vi "NMEA_PARSER.vi"(0 "previous partial sentence":string, 1 "sensor data":string, 3 "error in (no error)":errorcluster) -> (7 "remaining partial sentence":string, 8 "GPS data":T1 {"oldest read timestamp" format="%#_10g"; "latitude (deg)" format="%#_10g"; "longitude (deg)" format="%#_10g"}, 10 "error out":errorcluster)   [LabVIEW 2024]
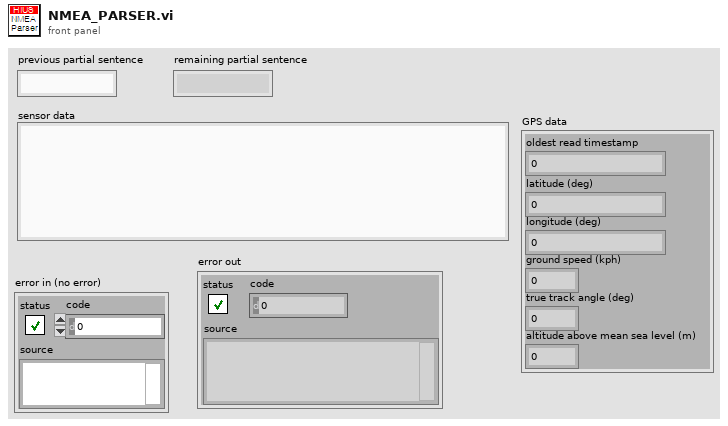
[diagram p1: front panel]
types:
  T1 = cluster{"oldest read timestamp":dbl, "latitude (deg)":dbl, "longitude (deg)":dbl, "ground speed (kph)":dbl, "true track angle (deg)":dbl, "altitude above mean sea level (m)":dbl}
  T2 = cluster{"oldest read timestamp":dbl, "latitude":dbl, "longitude":dbl, "speed over ground (kph)":dbl, "true track angle (deg)":dbl, "altitude above mean sea level":dbl}
  T3 = cluster{"time of fix":cluster{"included?":bool, "time (UTC)":dbl}, "status":cluster{"included?":bool, "value":u16}, "latitude":cluster{"included?":bool, "latitude (deg)":dbl}, "longitude":cluster{"included?":bool, "longitude (deg)":dbl}, "ground speed":cluster{"included?":bool, "speed (knots)":dbl}, "true track angle":cluster{"included?":bool, "angle (deg)":dbl}, "magnetic variation":cluster{"included?":bool, "variation (deg)":dbl}, "type of fix":cluster{"included?":bool, "mode":u16}}
  T4 = cluster{"time of fix":cluster{"included?":bool, "time (UTC)":dbl}, "latitude":cluster{"included?":bool, "latitude (deg)":dbl}, "longitude":cluster{"included?":bool, "longitude (deg)":dbl}, "ground speed (km/h)":cluster{"included?":bool, "speed (km/h)":dbl}, "ture track angle":cluster{"included?":bool, "angle (deg)":dbl}}
  T5 = cluster{"time of fix":cluster{"included?":bool, "time (UTC)":dbl}, "latitude":cluster{"included?":bool, "latitude (deg)":dbl}, "longitude":cluster{"included?":bool, "longitude (deg)":dbl}, "fix quality":cluster{"included?":bool, "quality":u16}, "number of satellites in view":cluster{"included?":bool, "number of satellites":i8}, "horizontal dilution of precision":cluster{"included?":bool, "horizontal DOP":dbl}, "altitude above mean sea level":cluster{"included?":bool, "altitude (m)":dbl}, "height of geoid above WGS84":cluster{"included?":bool, "height of geoid (m)":dbl}, "time since last DGPS update":cluster{"included?":bool, "time (s)":dbl}, "DGPS station ID number":cluster{"included?":bool, "station ID number":dbl}}
  T6 = cluster{"true track made good":cluster{"included?":bool, "true track made good (deg)":dbl}, "magnetic track made good":cluster{"included?":bool, "magnetic track made good (deg)":dbl}, "ground speed (knots)":cluster{"included?":bool, "speed (knots)":dbl}, "ground speed (km/h)":cluster{"included?":bool, "speed (km/h)":dbl}, "type of fix":cluster{"included?":bool, "mode":u16}}
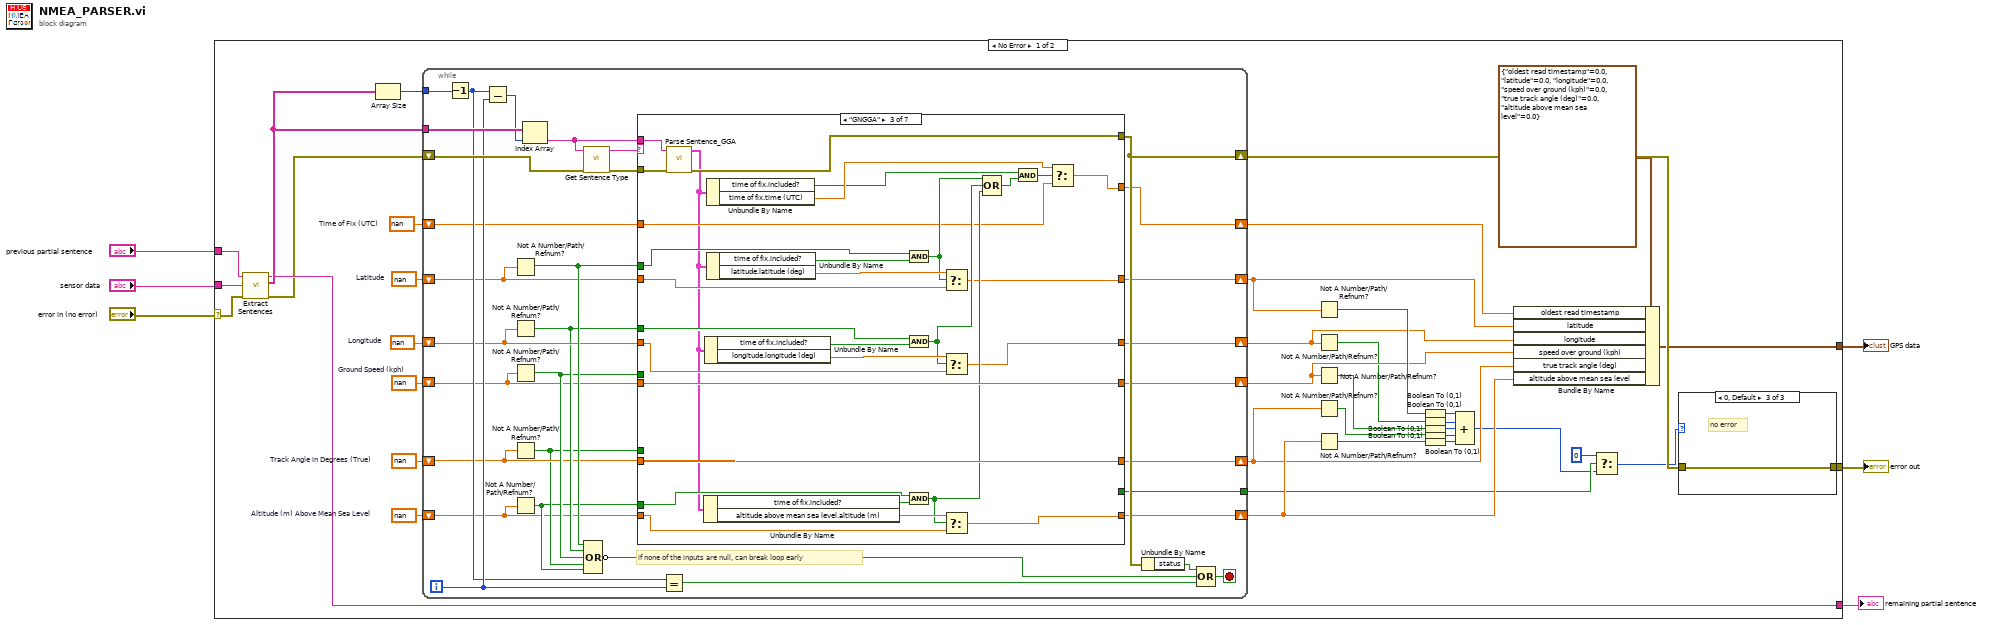
[diagram p0: block diagram]
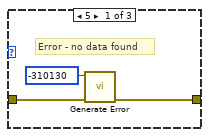
[diagram p2: hidden frame]
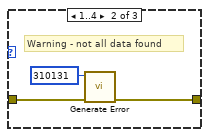
[diagram p3: hidden frame]
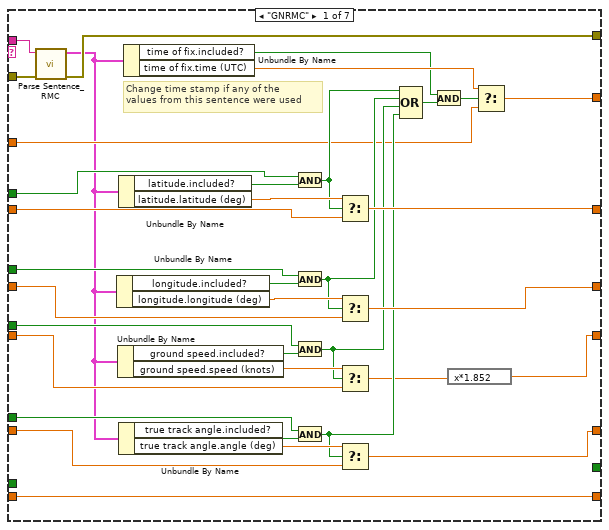
[diagram p4: hidden frame]
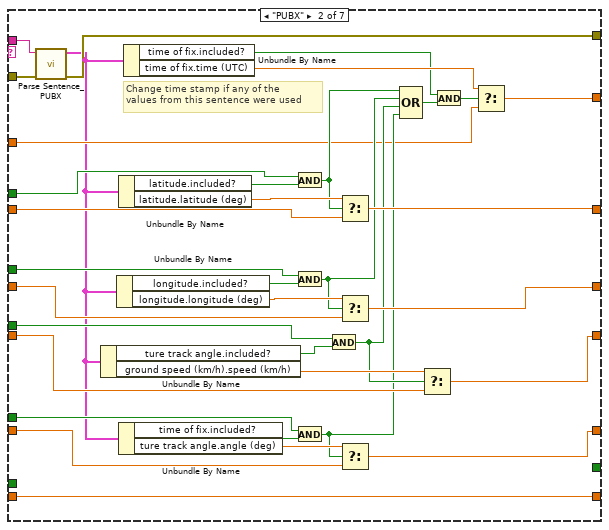
[diagram p5: hidden frame]
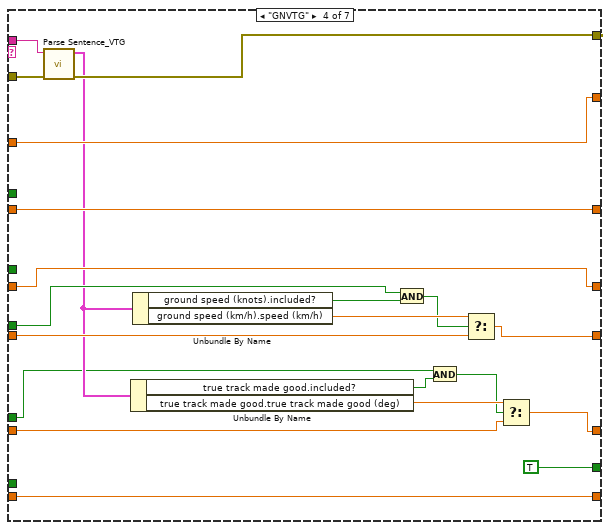
[diagram p6: hidden frame]
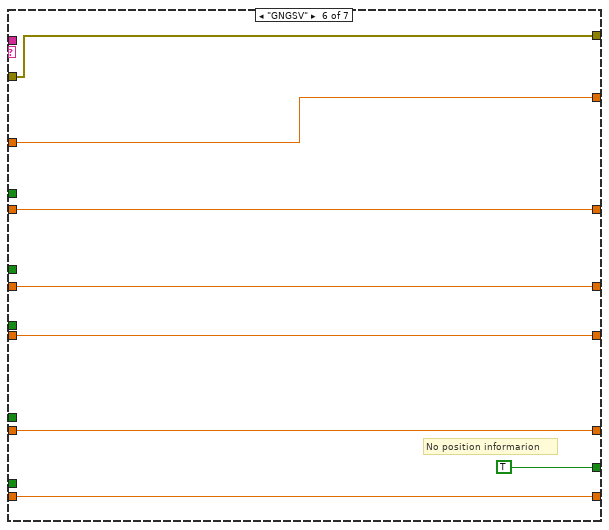
[diagram p8: hidden frame]
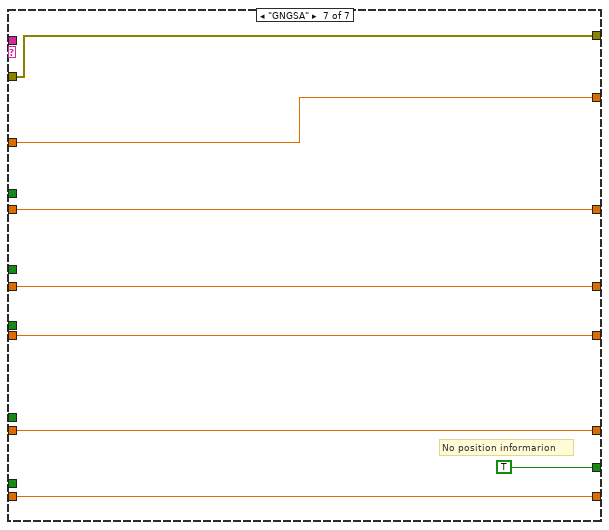
[diagram p9: hidden frame]
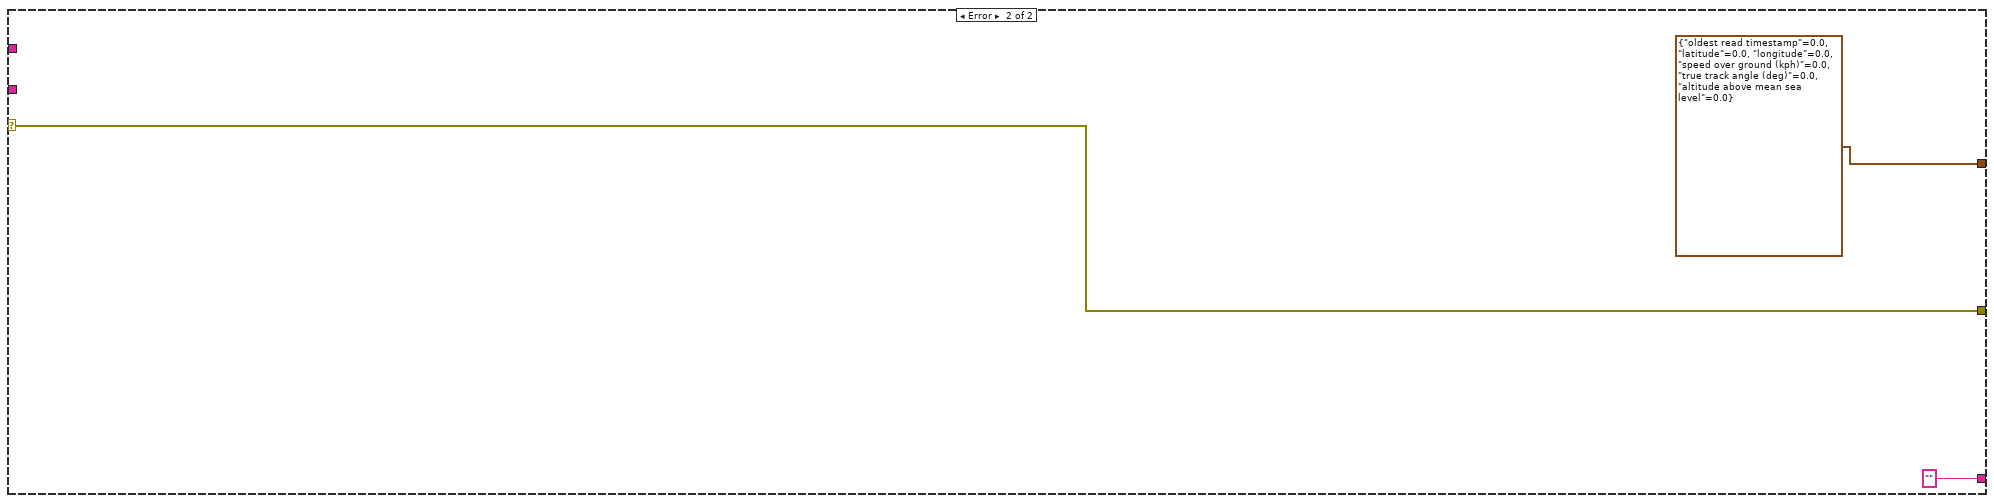
[diagram p10: hidden frame]
diagram:
  n1 = case shown="No Error" "error in (no error)" {
    selector: "error in (no error)" -> [w21 w230]
    tunnel: [w41 w230] -> w5
    tunnel: "sensor data" -> [w30 _]
    tunnel: "previous partial sentence" -> [w29 _]
    tunnel: [w28 T2 {"oldest read timestamp"=0.0, "latitude"=0.0, "longitude"=0.0, "speed over ground (kph)"=0.0, "true track angle (deg)"=0.0, "altitude above mean sea level"=0.0} ("GPS Data")] -> w4
    tunnel: [w22 "" ("After Last Sentence")] -> w3
    frame No Error {
      w34 = nan  # Altitude (m) Above Mean Sea Level
      w35 = nan  # Track Angle in Degrees (True)
      w32 = nan  # Ground Speed (kph)
      w36 = nan  # Longitude
      w37 = nan  # Latitude
      w38 = nan  # Time of Fix (UTC)
      n2 = call "Extract Sentences.vi"("error in (no error)"=w21, "sensor data"=w30, "previous partial sentence"=w29) -> ("error out"=w20:errorcluster, "complete sentences"=w40:string[], "remaining partial sentence"=w22:string)  [unwired: 4 in, 2 out]
      n3 = Array Size(array=w40) -> (size(s)=w39:i32)
      n4 = while {
        tunnel: w40 -> [w81]
        shift-right: [w77] -> w42
        shift-left: w20 -> [w79]
        shift-right: [w71] -> w43
        shift-left: w38 -> [w64]
        shift-right: [w69] -> w31
        shift-left: w37 -> [w62]
        shift-right: [w68] -> w15
        shift-left: w36 -> [w61]
        shift-right: [w76] -> w17
        shift-left: w35 -> [w57]
        shift-right: [w70] -> w18
        shift-left: w34 -> [w54]
        tunnel: w39 -> [w66]
        shift-right: [w67] -> w16
        shift-left: w32 -> [w58]
        tunnel: [w51] -> w10
        i -> [w74]
        stop <- w82 stop-if-true
        # "if none of the inputs are null, can break loop early"
        n5 = Decrement(x=w66) -> (x-1=w65:i32)
        n6 = Subtract(x=w65, y=w74) -> (x-y=w75:i32)
        n7 = Not A Number/Path/Refnum?(number/path/refnum=w62) -> (NaN/Path/Refnum?=w63:bool)
        n8 = Not A Number/Path/Refnum?(number/path/refnum=w61) -> (NaN/Path/Refnum?=w60:bool)
        n9 = Not A Number/Path/Refnum?(number/path/refnum=w58) -> (NaN/Path/Refnum?=w59:bool)
        n10 = Not A Number/Path/Refnum?(number/path/refnum=w57) -> (NaN/Path/Refnum?=w56:bool)
        n11 = Not A Number/Path/Refnum?(number/path/refnum=w54) -> (NaN/Path/Refnum?=w55:bool)
        n12 = Index Array(array=w81, index=w75) -> (element=w53:string)
        n13 = call "Get Sentence Type.vi"("error in (no error)"=w79, "sentence"=w53) -> ("error out"=w78:errorcluster, "sentence type"=w52:string)  [unwired: 7 in, 1 out]
        n14 = Compound Arithmetic op=OR(w63, w60, w59, w56, w55) -> (invert w72:bool)
        n15 = case shown="\"GNGGA\"" w52 {
          tunnel: w78 -> [w118 w153 w183 w204 w211 w219 w227]
          tunnel: [w117 w152 w181 w203 w211 w219 w227] -> w77
          tunnel: [w111 w146 w182 w185 w210 w218 w226] -> w76
          tunnel: w53 -> [w86 w120 w155 w196 _ _ _]
          tunnel: w64 -> [w91 w125 w158 w195 w209 w217 w225]
          tunnel: w62 -> [w98 w132 w163 w188 w207 w215 w223]
          tunnel: w61 -> [w103 w137 w169 w189 w206 w214 w222]
          tunnel: w57 -> [w112 w147 w182 w184 w210 w218 w226]
          tunnel: w54 -> [w116 w151 w177 w194 w208 w216 w224]
          tunnel: w63 -> [w100 w134 w164 _ _ _ _]
          tunnel: w60 -> [w105 w139 w171 _ _ _ _]
          tunnel: w59 -> [w107 w141 _ w190 _ _ _]
          tunnel: w56 -> [w114 w149 _ w186 _ _ _]
          tunnel: w55 -> [_ _ w176 _ _ _ _]
          tunnel: [w87 w121 w157 w195 w209 w217 w225] -> w71
          tunnel: [w116 w151 w174 w194 w208 w216 w224] -> w70
          tunnel: [w97 w131 w165 w188 w207 w215 w223] -> w69
          tunnel: [w83 w142 w180 w192 w205 w213 w221] -> w67
          tunnel: [w102 w136 w168 w189 w206 w214 w222] -> w68
          tunnel: w58 -> [w108 w143 w180 w191 w205 w213 w221]
          tunnel: [_ _ _ TRUE _ TRUE TRUE] -> w51
          frame "GNRMC" {
            # "Change time stamp if any of the\nvalues from this sentence were used"
            n16 = call "Parse Sentence_RMC.vi"("error in (no error)"=w118, "RMC sentence"=w86) -> ("error out"=w117:errorcluster, "RMC_Data"=w85:T3)  [unwired: 8 in]
            n17 = Unbundle By Name(w85) -> ("longitude.included?"=w106:bool, "longitude.longitude (deg)"=w104:dbl)
            n18 = Unbundle By Name(w85) -> ("ground speed.included?"=w110:bool, "ground speed.speed (knots)"=w109:dbl)
            n19 = Unbundle By Name(w85) -> ("latitude.included?"=w101:bool, "latitude.latitude (deg)"=w99:dbl)
            n20 = Unbundle By Name(w85) -> ("true track angle.included?"=w115:bool, "true track angle.angle (deg)"=w113:dbl)
            n21 = Unbundle By Name(w85) -> ("time of fix.included?"=w89:bool, "time of fix.time (UTC)"=w90:dbl)
            n22 = And(x=w100, y=w101) -> (x .and. y?=w96:bool)
            n23 = And(x=w105, y=w106) -> (x .and. y?=w95:bool)
            n24 = And(x=w107, y=w110) -> (x .and. y?=w94:bool)
            n25 = And(x=w114, y=w115) -> (x .and. y?=w93:bool)
            n26 = Select(t=w99, s=w96, f=w98) -> (s? t:f=w97:dbl)
            n27 = Select(t=w104, s=w95, f=w103) -> (s? t:f=w102:dbl)
            n28 = Select(t=w109, s=w94, f=w108) -> (s? t:f=w84:dbl)
            n29 = Select(t=w113, s=w93, f=w112) -> (s? t:f=w111:dbl)
            n30 = Compound Arithmetic op=OR(w96, w95, w94, w93) -> (w92:bool)
            n31 = And(x=w89, y=w92) -> (x .and. y?=w88:bool)
            n32 = expression code="x*1.852"(w84) -> (w83:dbl)
            n33 = Select(t=w90, s=w88, f=w91) -> (s? t:f=w87:dbl)
          }
          frame "PUBX" {
            # "Change time stamp if any of the\nvalues from this sentence were used"
            n34 = call "Parse Sentence_PUBX.vi"("error in (no error)"=w153, "PUBX sentence"=w120) -> ("error out"=w152:errorcluster, "PUBX_Data"=w119:T4)  [unwired: 8 in]
            n35 = Unbundle By Name(w119) -> ("ture track angle.included?"=w145:bool, "ground speed (km/h).speed (km/h)"=w144:dbl)
            n36 = Unbundle By Name(w119) -> ("longitude.included?"=w140:bool, "longitude.longitude (deg)"=w138:dbl)
            n37 = Unbundle By Name(w119) -> ("latitude.included?"=w135:bool, "latitude.latitude (deg)"=w133:dbl)
            n38 = Unbundle By Name(w119) -> ("time of fix.included?"=w150:bool, "ture track angle.angle (deg)"=w148:dbl)
            n39 = Unbundle By Name(w119) -> ("time of fix.included?"=w123:bool, "time of fix.time (UTC)"=w124:dbl)
            n40 = And(x=w134, y=w135) -> (x .and. y?=w130:bool)
            n41 = And(x=w139, y=w140) -> (x .and. y?=w129:bool)
            n42 = And(x=w149, y=w150) -> (x .and. y?=w127:bool)
            n43 = And(x=w141, y=w145) -> (x .and. y?=w128:bool)
            n44 = Select(t=w133, s=w130, f=w132) -> (s? t:f=w131:dbl)
            n45 = Select(t=w138, s=w129, f=w137) -> (s? t:f=w136:dbl)
            n46 = Select(t=w148, s=w127, f=w147) -> (s? t:f=w146:dbl)
            n47 = Compound Arithmetic op=OR(w130, w129, w128, w127) -> (w126:bool)
            n48 = Select(t=w144, s=w128, f=w143) -> (s? t:f=w142:dbl)
            n49 = And(x=w123, y=w126) -> (x .and. y?=w122:bool)
            n50 = Select(t=w124, s=w122, f=w125) -> (s? t:f=w121:dbl)
          }
          frame "GNGGA" {
            n51 = call "Parse Sentence_GGA.vi"("error in (no error)"=w183, "GGA sentence"=w155) -> ("error out"=w181:errorcluster, "GGA_Data"=w154:T5)  [unwired: 8 in]
            n52 = Unbundle By Name(w154) -> ("time of fix.included?"=w179:bool, "altitude above mean sea level.altitude (m)"=w178:dbl)
            n53 = Unbundle By Name(w154) -> ("time of fix.included?"=w173:bool, "longitude.longitude (deg)"=w172:dbl)
            n54 = Unbundle By Name(w154) -> ("time of fix.included?"=w160:bool, "time of fix.time (UTC)"=w161:dbl)
            n55 = Unbundle By Name(w154) -> ("time of fix.included?"=w167:bool, "latitude.latitude (deg)"=w166:dbl)
            n56 = And(x=w164, y=w167) -> (x .and. y?=w162:bool)
            n57 = And(x=w171, y=w173) -> (x .and. y?=w170:bool)
            n58 = And(x=w176, y=w179) -> (x .and. y?=w175:bool)
            n59 = Select(t=w166, s=w162, f=w163) -> (s? t:f=w165:dbl)
            n60 = Select(t=w172, s=w170, f=w169) -> (s? t:f=w168:dbl)
            n61 = Select(t=w178, s=w175, f=w177) -> (s? t:f=w174:dbl)
            n62 = Compound Arithmetic op=OR(w162, w170, w175) -> (w156:bool)
            n63 = And(x=w160, y=w156) -> (x .and. y?=w159:bool)
            n64 = Select(t=w161, s=w159, f=w158) -> (s? t:f=w157:dbl)
          }
          frame "GNVTG" {
            n65 = call "Parse Sentence_VTG.vi"("error in (no error)"=w204, "VTG sentence"=w196) -> ("error out"=w203:errorcluster, "VTG  data"=w187:T6)  [unwired: 8 in]
            n66 = Unbundle By Name(w187) -> ("true track made good.included?"=w199:bool, "true track made good.true track made good (deg)"=w198:dbl)
            n67 = Unbundle By Name(w187) -> ("ground speed (knots).included?"=w202:bool, "ground speed (km/h).speed (km/h)"=w201:dbl)
            n68 = And(x=w190, y=w202) -> (x .and. y?=w200:bool)
            n69 = And(x=w186, y=w199) -> (x .and. y?=w197:bool)
            n70 = Select(t=w201, s=w200, f=w191) -> (s? t:f=w192:dbl)
            n71 = Select(t=w198, s=w197, f=w184) -> (s? t:f=w185:dbl)
          }
          frame "", Default {
          }
          frame "GNGSV" {
            # "No position informarion"
          }
          frame "GNGSA" {
            # "No position informarion"
          }
        }
        n72 = Equal?(x=w65, y=w74) -> (x = y?=w80:bool)
        n73 = Unbundle By Name(w77) -> ("status"=w73:bool)
        n74 = Compound Arithmetic op=OR(w73, w72, w80) -> (w82:bool)
      }
      n75 = Not A Number/Path/Refnum?(number/path/refnum=w31) -> (NaN/Path/Refnum?=w19:bool)
      n76 = Not A Number/Path/Refnum?(number/path/refnum=w15) -> (NaN/Path/Refnum?=w14:bool)
      n77 = Not A Number/Path/Refnum?(number/path/refnum=w16) -> (NaN/Path/Refnum?=w13:bool)
      n78 = Not A Number/Path/Refnum?(number/path/refnum=w17) -> (NaN/Path/Refnum?=w12:bool)
      n79 = Not A Number/Path/Refnum?(number/path/refnum=w18) -> (NaN/Path/Refnum?=w11:bool)
      n80 = Boolean To (0,1)(Boolean=w19) -> (0, 1=w27:i16)
      n81 = Boolean To (0,1)(Boolean=w14) -> (0, 1=w26:i16)
      n82 = Boolean To (0,1)(Boolean=w13) -> (0, 1=w25:i16)
      n83 = Boolean To (0,1)(Boolean=w12) -> (0, 1=w24:i16)
      n84 = Boolean To (0,1)(Boolean=w11) -> (0, 1=w23:i16)
      n85 = Compound Arithmetic op=ADD(w27, w26, w25, w24, w23) -> (w9:i16)
      n86 = Bundle By Name(cluster=T2 {"oldest read timestamp"=0.0, "latitude"=0.0, "longitude"=0.0, "speed over ground (kph)"=0.0, "true track angle (deg)"=0.0, "altitude above mean sea level"=0.0} ("GPS Data"), "oldest read timestamp"=w43, "latitude"=w31, "longitude"=w15, "speed over ground (kph)"=w16, "true track angle (deg)"=w17, "altitude above mean sea level"=w18) -> (w28:T2)
      n87 = Select(t=i16 0, s=w10, f=w9) -> (s? t:f=w8:i16)
      n88 = case shown="0, Default" w8 {
        tunnel: w42 -> [w46 w48 w50]
        tunnel: [w45 w47 w50] -> w41
        frame 5 {
          # "Error - no data found"
          n89 = call "Generate Error.vi"("error in (no error)"=w46, "code"=-310130) -> ("error out"=w45:errorcluster)  [unwired: 9 in]
        }
        frame 1..4 {
          # "Warning - not all data found"
          n90 = call "Generate Error.vi"("error in (no error)"=w48, "code"=310131) -> ("error out"=w47:errorcluster)  [unwired: 9 in]
        }
        frame 0, Default {
          # "no error"
        }
      }
    }
    frame Error {
    }
  }
  "error out" <- w5
  "remaining partial sentence" <- w3
  "GPS data" <- w4
